vi "Get Active Project Name.vi"(8 "error in":errorcluster) -> (0 "error out":errorcluster, 2 "Project Name":string, 3 "My Computer Target":refnum<vi>, 5 "Project":refnum<vi>)   [LabVIEW 2019, in "Panther Dashboard.lvlib"]
uses:
  Panther Dashboard.lvlib
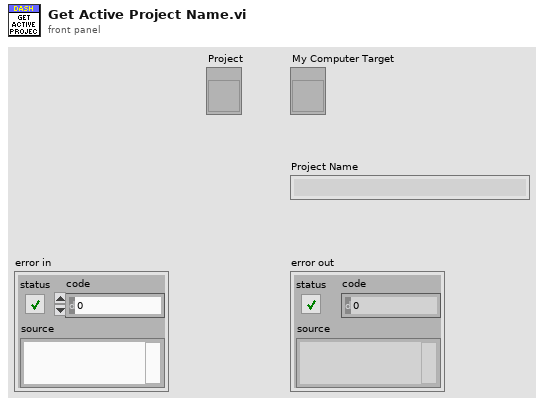
[diagram p1: front panel]
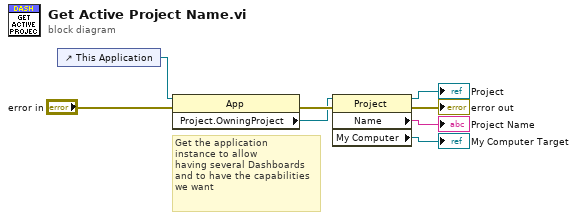
[diagram p0: block diagram]
diagram:
  # "Get the application\ninstance to allow\nhaving several Dashboards\nand to have the capabilities\nwe want"
  n1 = control-ref of="This Application"() -> (w4:refnum<vi>)
  n2 = property class="App"(reference=w4, error in="error in") -> (error out=w7:errorcluster, "Project.OwningProject"=w5:refnum<vi>)  [unwired: 1 out]
  n3 = property class="Project"(reference=w5, error in=w7) -> (reference out=→"Project":refnum<vi>, error out=→"error out":errorcluster, "Name"=→"Project Name":string, "My Computer"=→"My Computer Target":refnum<vi>)
